vi "pp2_DAQwriteAudio.vi"(5 "Daq config In":T1={"Sound AO"="Dev2/ao0", "Shock intesity AO"="Dev1/ao1", "Code_LED DO"="Dev1/port1:2", "Switch DI"="Dev1/port0/line0:1", "Webcam"="cam0", "Sound AO task"="", "Sound card task"=0, "Shock intensity AO task"="", "Code_LED DO task"="", "Switch DI task"="", "AO <=> Sound card"=FALSE, "Sound card"=0, "sample rate"=8000.0, "Variable shock"=FALSE, "Webcam on"=FALSE, "Tone gate PFI"="/Dev1/PFI1", "Waveform memo"={"t0"=timestamp(0 s since 1904-01-01), "dt"=1.0, "Y"=[]}} {"sample rate" min=8000.0; "Sound card task" format="%.0x"}, 7 "Waveform":waveform(dbl), 11 "error in (no error)":errorcluster) -> (6 "Daq config Out":T1={"Sound AO"="Dev2/ao0", "Shock intesity AO"="Dev1/ao1", "Code_LED DO"="Dev1/port1:2", "Switch DI"="Dev1/port0/line0:1", "Webcam"="cam0", "Sound AO task"="", "Sound card task"=0, "Shock intensity AO task"="", "Code_LED DO task"="", "Switch DI task"="", "AO <=> Sound card"=FALSE, "Sound card"=0, "sample rate"=8000.0, "Variable shock"=FALSE, "Webcam on"=FALSE, "Tone gate PFI"="/Dev1/PFI1", "Waveform memo"={"t0"=timestamp(0 s since 1904-01-01), "dt"=1.0, "Y"=[]}} {"sample rate" min=8000.0; "Sound card task" format="%.0x"}, 15 "error out":errorcluster)   [LabVIEW 2013]
uses:
  pp2_CTL_DaqConfig.ctl
  <vilib>/userdefined/High Color/IMAQdx.ctl
  <vilib>/sound2/lvsound2.llb/Sound Output Task ID.ctl
  <vilib>/DAQmx/create/channels.llb/DAQmx Create Channel (AO-Voltage-Basic).vi
  <vilib>/DAQmx/configure/timing.llb/DAQmx Timing (Use Waveform).vi
  <vilib>/DAQmx/write.llb/DAQmx Write (Analog Wfm 1Chan NSamp).vi
  <resource>/objmgr/daqmx.rc
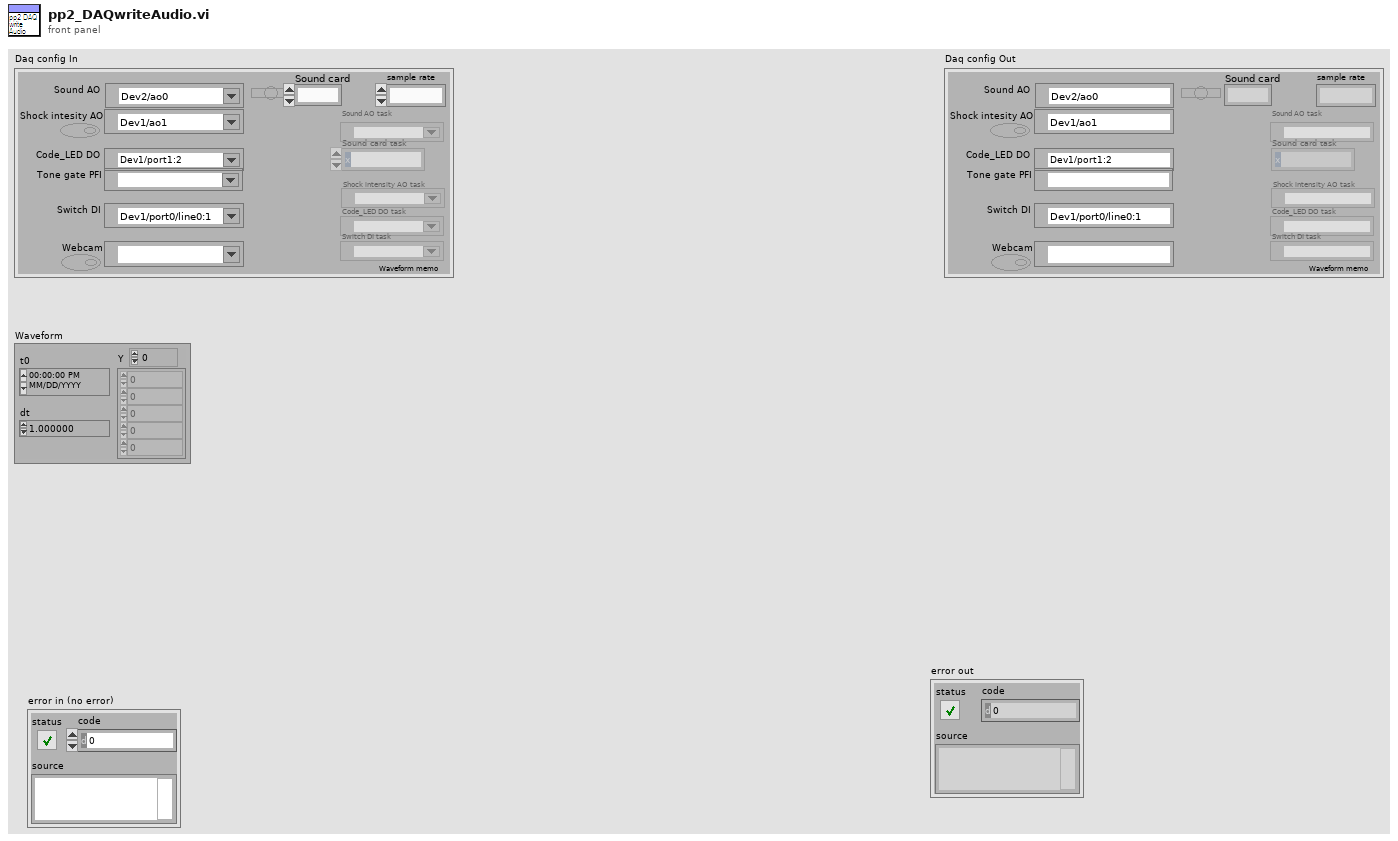
[diagram p1: front panel]
types:
  T1 = typedef "pp2_CTL_DaqConfig.ctl" = cluster{"Sound AO":tag, "Shock intesity AO":tag, "Code_LED DO":tag, "Switch DI":tag, "Webcam":T2, "Sound AO task":refnum<k21>, "Sound card task":T3, "Shock intensity AO task":refnum<k21>, "Code_LED DO task":refnum<k21>, "Switch DI task":refnum<k21>, "AO <=> Sound card":bool, "Sound card":u32, "sample rate":dbl, "Variable shock":bool, "Webcam on":bool, "Tone gate PFI":tag, "Waveform memo":waveform(dbl)}
  T2 = typedef "IMAQdx.ctl" = refnum<k21>
  T3 = typedef "Sound Output Task ID.ctl" = u32
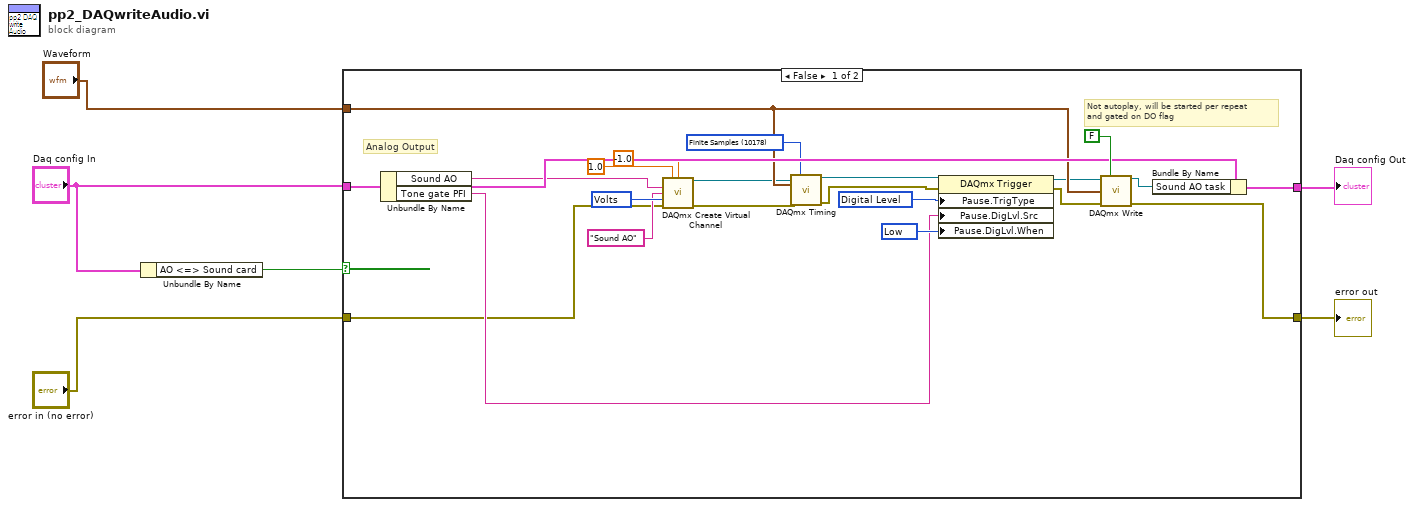
[diagram p0: block diagram]
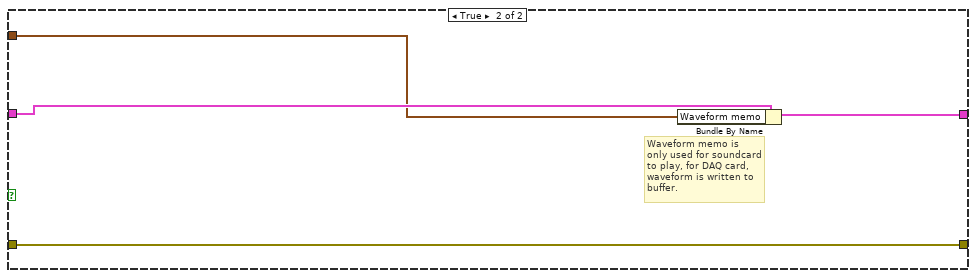
[diagram p2: hidden frame]
diagram:
  n1 = Unbundle By Name("Daq config In") -> ("AO <=> Sound card"=w6:bool)
  n2 = case shown="False" w6 {
    tunnel: "Daq config In" -> [w27 w31]
    tunnel: [w26 w32] -> w3
    tunnel: "error in (no error)" -> [w7 w29]
    tunnel: [w24 w29] -> w2
    tunnel: "Waveform" -> [w22 w30]
    frame False {
      w14 = 10348 items=["Volts"=10348, "From Custom Scale"=10065] ("units")
      w20 = 10214 items=["High"=10192, "Low"=10214] ("Pause.DigLvl.When")
      w21 = 10152 items=["Analog Level"=10101, "Analog Window"=10103, "Digital Level"=10152, "Digital Pattern"=10398, "None"=10230] ("Pause.TrigType")
      w23 = 10178 items=["Finite Samples"=10178, "Continuous Samples"=10123, "Hardware Timed Single Point"=12522] ("sample mode")
      # "Not autoplay, will be started per repeat\nand gated on DO flag"
      # "Analog Output"
      n3 = Unbundle By Name(w27) -> ("Sound AO"=w8:tag, "Tone gate PFI"=w15:tag)
      n4 = call-poly <vilib>:"DAQmx Create Virtual Channel.vi"("maximum value"=1.0, "minimum value"=-1.0, "physical channels"=w8, "name to assign"="Sound AO", "units"=w14, "error in"=w7) -> ("task out"=w10:refnum<k21>, "error out"=w9:errorcluster)  [unwired: 8 in]
      n5 = call-poly <vilib>:"DAQmx Timing.vi"("task/channels in"=w10, "sample mode"=w23, "waveform"=w22, "error in"=w9) -> ("task out"=w19:refnum<k21>, "error out"=w18:errorcluster)  [unwired: 10 in]
      n6 = property class="DAQmx Trigger"(reference=w19, error in=w18, "Pause.TrigType"=w21, "Pause.DigLvl.Src"=w15, "Pause.DigLvl.When"=w20) -> (reference out=w16:refnum<k21>, error out=w17:errorcluster)
      n7 = call-poly <vilib>:"DAQmx Write.vi"("task/channels in"=w16, "auto start"=FALSE, "data"=w22, "error in"=w17) -> ("task out"=w25:refnum<k21>, "error out"=w24:errorcluster)  [unwired: 9 in, 1 out]
      n8 = Bundle By Name(cluster=w27, "Sound AO task"=w25) -> (w26:T1)
    }
    frame True {
      # "Waveform memo is\nonly used for soundcard\nto play, for DAQ card,\nwaveform is written to\nbuffer."
      n9 = Bundle By Name(cluster=w31, "Waveform memo"=w30) -> (w32:T1)
    }
  }
  "Daq config Out" <- w3
  "error out" <- w2
